vi "Read Module Menu Name.vi"(8 "error in":errorcluster, 11 "tag bus configurable plugin editor node in":refnum<class "fixed channel tag bus module editor node.lvclass">) -> (0 "error out":errorcluster, 2 "Menu Name":string, 3 "tag bus configurable plugin editor node out":refnum<class "fixed channel tag bus module editor node.lvclass">)   [LabVIEW 2013, in "fixed channel tag bus module editor node.lvclass"]
uses:
  fixed channel tag bus module editor node.lvclass
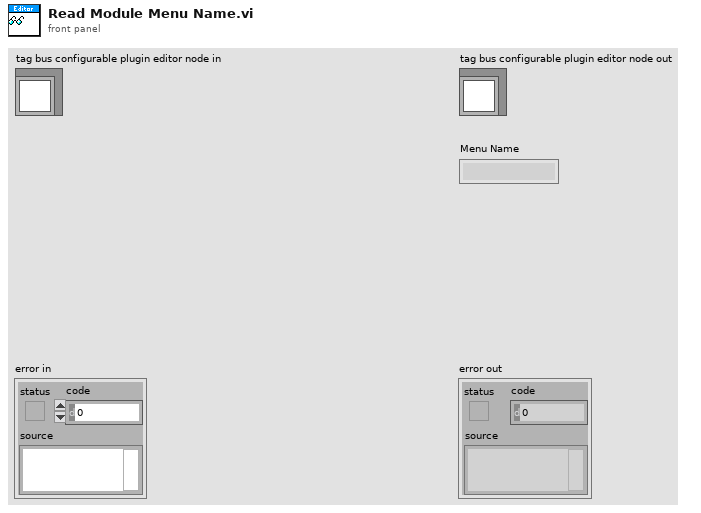
[diagram p1: front panel]
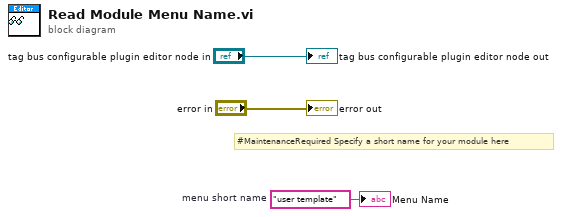
[diagram p0: block diagram]
diagram:
  w1 = "user template"  # menu short name
  # "#MaintenanceRequired Specify a short name for your module here"
  "error out" <- "error in"
  "tag bus configurable plugin editor node out" <- "tag bus configurable plugin editor node in"
  "Menu Name" <- w1
